vi "MEM Graph Holder.vi"(1 "Action(GET)":T5(ring), 7 "Mem Graph Ctl In":T1={"Chart Visible Time selector"=enum."1 minute", "Plot G1 L1"={"Var Tag"=0, "Color"=0, "Line Width"=0}, "Plot G1 L2"={"Var Tag"=0, "Color"=0, "Line Width"=0}, "Plot G1 R1"={"Var Tag"=0, "Color"=0, "Line Width"=0}, "Plot G1 R2"={"Var Tag"=0, "Color"=0, "Line Width"=0}, "Plot G2 L1"={"Var Tag"=0, "Color"=0, "Line Width"=0}, "Plot G2 L2"={"Var Tag"=0, "Color"=0, "Line Width"=0}, "Plot G2 R1"={"Var Tag"=0, "Color"=0, "Line Width"=0}, "Plot G2 R2"={"Var Tag"=0, "Color"=0, "Line Width"=0}, "G1 Y scale 0"={"Maximum"=0.0, "Minimum"=0.0, "Autoscaling"=0}, "G1 Y scale 1"={"Maximum"=0.0, "Minimum"=0.0, "Autoscaling"=0}, "G2 Y scale 0"={"Maximum"=0.0, "Minimum"=0.0, "Autoscaling"=0}, "G2 Y scale 1"={"Maximum"=0.0, "Minimum"=0.0, "Autoscaling"=0}} {"Plot G2 R2"."Line Width" items=["0", "1", "2", "3", "4", "5"]; "Plot G2 R2"."Var Tag" items=["", "Wire Length", "Wire Tension", "Wire Speed", "Topside Voltage", "Tool Head Voltage", "Current", "Resistance"]; "Plot G2 R1"."Line Width" items=["0", "1", "2", "3", "4", "5"]; "Plot G2 R1"."Var Tag" items=["", "Wire Length", "Wire Tension", "Wire Speed", "Topside Voltage", "Tool Head Voltage", "Current", "Resistance"]; "Plot G2 L2"."Line Width" items=["0", "1", "2", "3", "4", "5"]; "Plot G2 L2"."Var Tag" items=["", "Wire Length", "Wire Tension", "Wire Speed", "Topside Voltage", "Tool Head Voltage", "Current", "Resistance"]; "Plot G2 L1"."Line Width" items=["0", "1", "2", "3", "4", "5"]; "Plot G2 L1"."Var Tag" items=["", "Wire Length", "Wire Tension", "Wire Speed", "Topside Voltage", "Tool Head Voltage", "Current", "Resistance"]; "Plot G1 L1"."Line Width" items=["0", "1", "2", "3", "4", "5"]; "Plot G1 L1"."Var Tag" items=["", "Wire Length", "Wire Tension", "Wire Speed", "Topside Voltage", "Tool Head Voltage", "Current", "Resistance"]; "Plot G1 L2"."Line Width" items=["0", "1", "2", "3", "4", "5"]; "Plot G1 L2"."Var Tag" items=["", "Wire Length", "Wire Tension", "Wire Speed", "Topside Voltage", "Tool Head Voltage", "Current", "Resistance"]; "Plot G1 R2"."Line Width" items=["0", "1", "2", "3", "4", "5"]; "Plot G1 R2"."Var Tag" items=["", "Wire Length", "Wire Tension", "Wire Speed", "Topside Voltage", "Tool Head Voltage", "Current", "Resistance"]; "Plot G1 R1"."Line Width" items=["0", "1", "2", "3", "4", "5"]; "Plot G1 R1"."Var Tag" items=["", "Wire Length", "Wire Tension", "Wire Speed", "Topside Voltage", "Tool Head Voltage", "Current", "Resistance"]}, 11 "error in (no error)":errorcluster) -> (8 "Mem Graph Ctl Out":T1={"Chart Visible Time selector"=enum."1 minute", "Plot G1 L1"={"Var Tag"=0, "Color"=0, "Line Width"=0}, "Plot G1 L2"={"Var Tag"=0, "Color"=0, "Line Width"=0}, "Plot G1 R1"={"Var Tag"=0, "Color"=0, "Line Width"=0}, "Plot G1 R2"={"Var Tag"=0, "Color"=0, "Line Width"=0}, "Plot G2 L1"={"Var Tag"=0, "Color"=0, "Line Width"=0}, "Plot G2 L2"={"Var Tag"=0, "Color"=0, "Line Width"=0}, "Plot G2 R1"={"Var Tag"=0, "Color"=0, "Line Width"=0}, "Plot G2 R2"={"Var Tag"=0, "Color"=0, "Line Width"=0}, "G1 Y scale 0"={"Maximum"=0.0, "Minimum"=0.0, "Autoscaling"=0}, "G1 Y scale 1"={"Maximum"=0.0, "Minimum"=0.0, "Autoscaling"=0}, "G2 Y scale 0"={"Maximum"=0.0, "Minimum"=0.0, "Autoscaling"=0}, "G2 Y scale 1"={"Maximum"=0.0, "Minimum"=0.0, "Autoscaling"=0}} {"Plot G2 R2"."Line Width" items=["0", "1", "2", "3", "4", "5"]; "Plot G2 R2"."Var Tag" items=["", "Wire Length", "Wire Tension", "Wire Speed", "Topside Voltage", "Tool Head Voltage", "Current", "Resistance"]; "Plot G2 R1"."Line Width" items=["0", "1", "2", "3", "4", "5"]; "Plot G2 R1"."Var Tag" items=["", "Wire Length", "Wire Tension", "Wire Speed", "Topside Voltage", "Tool Head Voltage", "Current", "Resistance"]; "Plot G2 L2"."Line Width" items=["0", "1", "2", "3", "4", "5"]; "Plot G2 L2"."Var Tag" items=["", "Wire Length", "Wire Tension", "Wire Speed", "Topside Voltage", "Tool Head Voltage", "Current", "Resistance"]; "Plot G2 L1"."Line Width" items=["0", "1", "2", "3", "4", "5"]; "Plot G2 L1"."Var Tag" items=["", "Wire Length", "Wire Tension", "Wire Speed", "Topside Voltage", "Tool Head Voltage", "Current", "Resistance"]; "Plot G1 L1"."Line Width" items=["0", "1", "2", "3", "4", "5"]; "Plot G1 L1"."Var Tag" items=["", "Wire Length", "Wire Tension", "Wire Speed", "Topside Voltage", "Tool Head Voltage", "Current", "Resistance"]; "Plot G1 L2"."Line Width" items=["0", "1", "2", "3", "4", "5"]; "Plot G1 L2"."Var Tag" items=["", "Wire Length", "Wire Tension", "Wire Speed", "Topside Voltage", "Tool Head Voltage", "Current", "Resistance"]; "Plot G1 R2"."Line Width" items=["0", "1", "2", "3", "4", "5"]; "Plot G1 R2"."Var Tag" items=["", "Wire Length", "Wire Tension", "Wire Speed", "Topside Voltage", "Tool Head Voltage", "Current", "Resistance"]; "Plot G1 R1"."Line Width" items=["0", "1", "2", "3", "4", "5"]; "Plot G1 R1"."Var Tag" items=["", "Wire Length", "Wire Tension", "Wire Speed", "Topside Voltage", "Tool Head Voltage", "Current", "Resistance"]}, 15 "error out":errorcluster)   [LabVIEW 2011]
uses:
  Mem Graph Ctl Custer.ctl
  GUI/Shart Time Selector.ctl
  GUI/Graph/Plot selector.ctl
  GUI/Graph/Y scale cluster.ctl
  <vilib>/Utility/VariantDataType/VariantType.lvlib
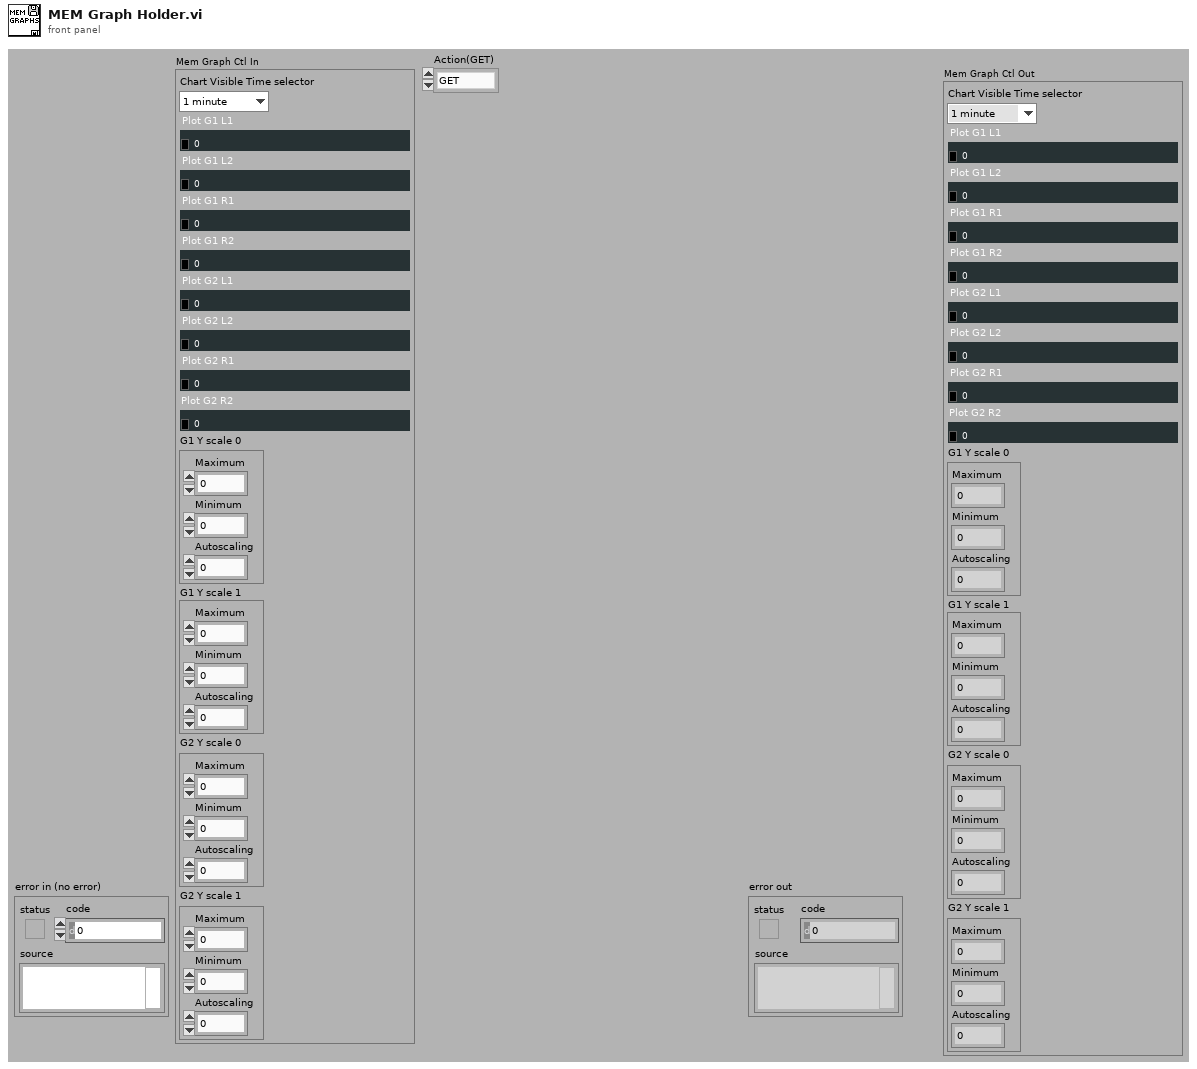
[diagram p1: front panel]
types:
  T1 = typedef "Mem Graph Ctl Custer.ctl" = cluster{"Chart Visible Time selector":T2, "Plot G1 L1":T3, "Plot G1 L2":T3, "Plot G1 R1":T3, "Plot G1 R2":T3, "Plot G2 L1":T3, "Plot G2 L2":T3, "Plot G2 R1":T3, "Plot G2 R2":T3, "G1 Y scale 0":T4, "G1 Y scale 1":T4, "G2 Y scale 0":T4, "G2 Y scale 1":T4}
  T2 = typedef "Shart Time Selector.ctl" = enum16{"10 Seconds", "1 minute", "5 minutes", "10 minutes", "30 minutes", "1 Hour"}
  T3 = typedef "Plot selector.ctl" = cluster{"Var Tag":u16, "Color":u32, "Line Width":u16}
  T4 = typedef "Y scale cluster.ctl" = cluster{"Maximum":dbl, "Minimum":dbl, "Autoscaling":i32}
  T5 = enum16{"GET", "SET", "Get from Ini", "Put in Ini"}
  T6 = typedef "List of tools.ctl" = enum16{"Stroker", "Driller", "Tractor"}
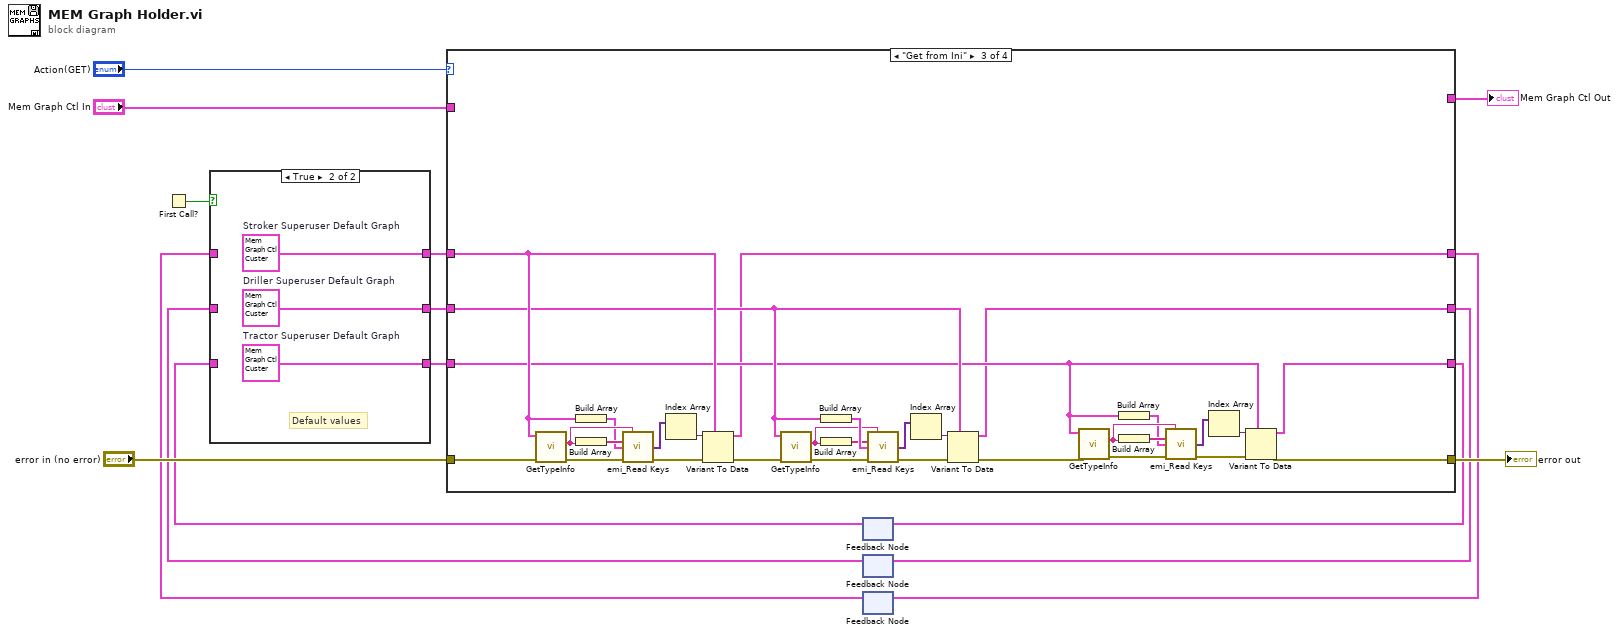
[diagram p0: block diagram]
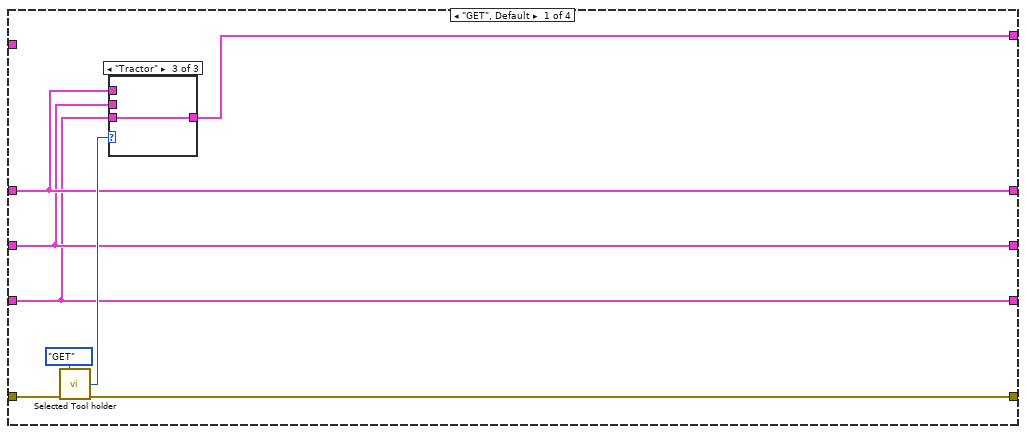
[diagram p3: hidden frame]
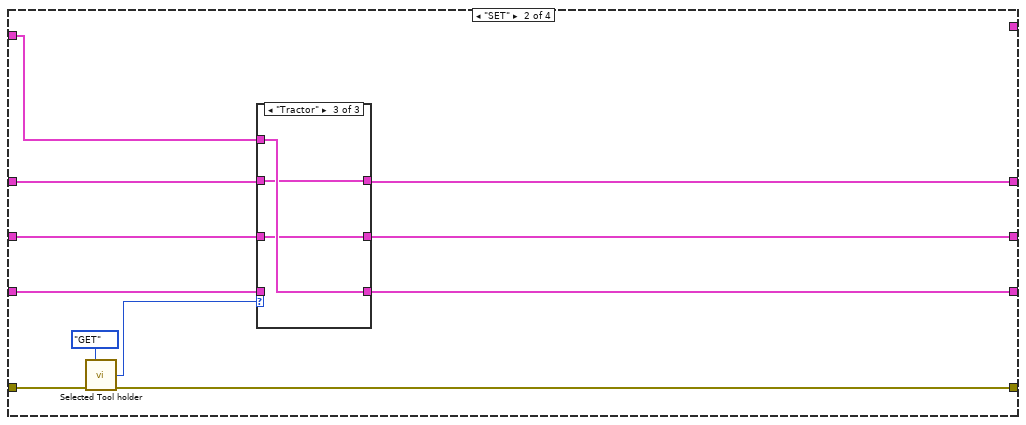
[diagram p6: hidden frame]
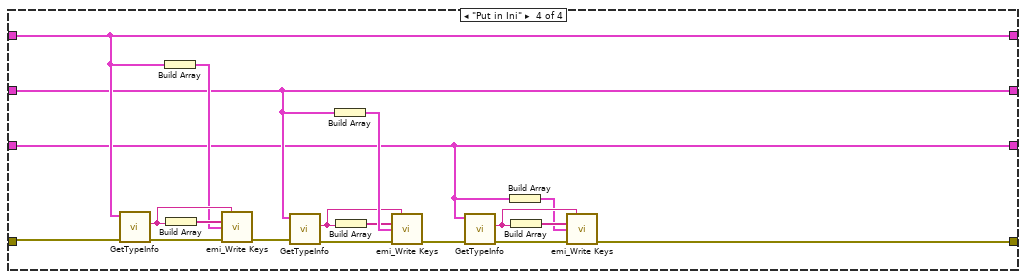
[diagram p9: hidden frame]
diagram:
  n1 = First Call?() -> (First Call?: T/F=w14:bool)
  n2 = feedback #1() -> (w1:T1)  [unwired: 1 in]
  n3 = feedback #2() -> (w2:T1)  [unwired: 1 in]
  n4 = feedback #3() -> (w3:T1)  [unwired: 1 in]
  n5 = case shown="True" w14 {
    tunnel: w3 -> [w18 _]
    tunnel: [w18 w21] -> w9
    tunnel: [w17 w20] -> w8
    tunnel: [w16 w19] -> w7
    tunnel: w2 -> [w17 _]
    tunnel: w1 -> [w16 _]
    frame False {
    }
    frame True {
      w19 = T1 {"Chart Visible Time selector"=enum."1 minute", "Plot G1 L1"={"Var Tag"=0, "Color"=16711680, "Line Width"=2}, "Plot G1 L2"={"Var Tag"=0, "Color"=16776960, "Line Width"=2}, "Plot G1 R1"={"Var Tag"=0, "Color"=16860, "Line Width"=2}, "Plot G1 R2"={"Var Tag"=0, "Color"=6618880, "Line Width"=2}, "Plot G2 L1"={"Var Tag"=0, "Color"=16711680, "Line Width"=2}, "Plot G2 L2"={"Var Tag"=0, "Color"=16776960, "Line Width"=2}, "Plot G2 R1"={"Var Tag"=0, "Color"=16860, "Line Width"=2}, "Plot G2 R2"={"Var Tag"=0, "Color"=6618880, "Line Width"=2}, "G1 Y scale 0"={"Maximum"=1.0, "Minimum"=-1.0, "Autoscaling"=0}, "G1 Y scale 1"={"Maximum"=1.0, "Minimum"=-1.0, "Autoscaling"=0}, "G2 Y scale 0"={"Maximum"=1.0, "Minimum"=-1.0, "Autoscaling"=0}, "G2 Y scale 1"={"Maximum"=1.0, "Minimum"=-1.0, "Autoscaling"=0}}  # Tractor Superuser Default Graph
      w20 = T1 {"Chart Visible Time selector"=enum."1 minute", "Plot G1 L1"={"Var Tag"=0, "Color"=16711680, "Line Width"=2}, "Plot G1 L2"={"Var Tag"=0, "Color"=16776960, "Line Width"=2}, "Plot G1 R1"={"Var Tag"=0, "Color"=16860, "Line Width"=2}, "Plot G1 R2"={"Var Tag"=0, "Color"=6618880, "Line Width"=2}, "Plot G2 L1"={"Var Tag"=0, "Color"=16711680, "Line Width"=2}, "Plot G2 L2"={"Var Tag"=0, "Color"=16776960, "Line Width"=2}, "Plot G2 R1"={"Var Tag"=0, "Color"=16860, "Line Width"=2}, "Plot G2 R2"={"Var Tag"=0, "Color"=6618880, "Line Width"=2}, "G1 Y scale 0"={"Maximum"=1.0, "Minimum"=-1.0, "Autoscaling"=0}, "G1 Y scale 1"={"Maximum"=1.0, "Minimum"=-1.0, "Autoscaling"=0}, "G2 Y scale 0"={"Maximum"=1.0, "Minimum"=-1.0, "Autoscaling"=0}, "G2 Y scale 1"={"Maximum"=1.0, "Minimum"=-1.0, "Autoscaling"=0}}  # Driller Superuser Default Graph
      w21 = T1 {"Chart Visible Time selector"=enum."1 minute", "Plot G1 L1"={"Var Tag"=0, "Color"=16711680, "Line Width"=2}, "Plot G1 L2"={"Var Tag"=0, "Color"=16776960, "Line Width"=2}, "Plot G1 R1"={"Var Tag"=0, "Color"=16860, "Line Width"=2}, "Plot G1 R2"={"Var Tag"=0, "Color"=6618880, "Line Width"=2}, "Plot G2 L1"={"Var Tag"=0, "Color"=16711680, "Line Width"=2}, "Plot G2 L2"={"Var Tag"=0, "Color"=16776960, "Line Width"=2}, "Plot G2 R1"={"Var Tag"=0, "Color"=16860, "Line Width"=2}, "Plot G2 R2"={"Var Tag"=0, "Color"=6618880, "Line Width"=2}, "G1 Y scale 0"={"Maximum"=1.0, "Minimum"=-1.0, "Autoscaling"=0}, "G1 Y scale 1"={"Maximum"=1.0, "Minimum"=-1.0, "Autoscaling"=0}, "G2 Y scale 0"={"Maximum"=1.0, "Minimum"=-1.0, "Autoscaling"=0}, "G2 Y scale 1"={"Maximum"=1.0, "Minimum"=-1.0, "Autoscaling"=0}}  # Stroker Superuser Default Graph
      # "Default values"
    }
  }
  n6 = case shown="\"Get from Ini\"" "Action(GET)" {
    tunnel: "error in (no error)" -> [w28 w35 w60 w88]
    tunnel: [w26 w34 w59 w87] -> w12
    tunnel: [w22 _ _ _] -> w10
    tunnel: "Mem Graph Ctl In" -> [_ w43 _ _]
    tunnel: w9 -> [w25 w42 w58 w86]
    tunnel: w8 -> [w24 w41 w57 w85]
    tunnel: w7 -> [w23 w40 w56 w84]
    tunnel: [w25 w37 w55 w86] -> w4
    tunnel: [w24 w38 w54 w85] -> w5
    tunnel: [w23 w39 w53 w84] -> w6
    frame "GET", Default {
      n7 = call "Selected Tool holder.vi"("Action(GET)"=enum16{"GET", "SET"}."GET", "error in (no error)"=w28) -> ("Tool out"=w27:T6, "error out"=w26:errorcluster)  [unwired: 12 in]
      n8 = case shown="\"Tractor\"" w27 {
        tunnel: w25 -> [w30 _ _]
        tunnel: w24 -> [_ w31 _]
        tunnel: w23 -> [_ _ w32]
        tunnel: [w30 w31 w32] -> w22
        frame "Stroker", Default {
        }
        frame "Driller" {
        }
        frame "Tractor" {
        }
      }
    }
    frame "SET" {
      n9 = call "Selected Tool holder.vi"("Action(GET)"=enum16{"GET", "SET"}."GET", "error in (no error)"=w35) -> ("Tool out"=w33:T6, "error out"=w34:errorcluster)  [unwired: 12 in]
      n10 = case shown="\"Tractor\"" w33 {
        tunnel: w43 -> [w46 w47 w52]
        tunnel: w40 -> [w44 w49 _]
        tunnel: w41 -> [w45 _ w51]
        tunnel: w42 -> [_ w48 w50]
        tunnel: [w45 w47 w51] -> w38
        tunnel: [w44 w49 w52] -> w39
        tunnel: [w46 w48 w50] -> w37
        frame "Stroker", Default {
        }
        frame "Driller" {
        }
        frame "Tractor" {
        }
      }
    }
    frame "Get from Ini" {
      n11 = call <vilib>:"GetTypeInfo.vi"("error in (no error)"=w60, "Variant"=w58) -> ("error out"=w64:errorcluster, "Name"=w65:string)  [unwired: 5 in, 3 out]
      n12 = Build Array(w58) -> (w61:T1[])
      n13 = Build Array(w65) -> (w62:string[])
      n14 = call "emi_Read Keys.vi"("Section"=w65, "Key Names"=w62, "Types/Defaults"=w61, "error in (no error)"=w64) -> ("Values"=w63:variant[], "error out"=w67:errorcluster)  [unwired: 9 in, 1 out]
      n15 = Index Array(array=w63) -> (element=w66:variant)  [unwired: 1 in]
      n16 = Variant To Data(error in=w67, type=w58, Variant=w66) -> (data=w55:T1, error out=w75:errorcluster)
      n17 = call <vilib>:"GetTypeInfo.vi"("error in (no error)"=w75, "Variant"=w57) -> ("error out"=w71:errorcluster, "Name"=w70:string)  [unwired: 5 in, 3 out]
      n18 = Build Array(w57) -> (w74:T1[])
      n19 = Build Array(w70) -> (w73:string[])
      n20 = call "emi_Read Keys.vi"("Section"=w70, "Key Names"=w73, "Types/Defaults"=w74, "error in (no error)"=w71) -> ("Values"=w72:variant[], "error out"=w68:errorcluster)  [unwired: 9 in, 1 out]
      n21 = Index Array(array=w72) -> (element=w69:variant)  [unwired: 1 in]
      n22 = Variant To Data(error in=w68, type=w57, Variant=w69) -> (data=w54:T1, error out=w83:errorcluster)
      n23 = call <vilib>:"GetTypeInfo.vi"("error in (no error)"=w83, "Variant"=w56) -> ("error out"=w79:errorcluster, "Name"=w80:string)  [unwired: 5 in, 3 out]
      n24 = Build Array(w56) -> (w76:T1[])
      n25 = Build Array(w80) -> (w77:string[])
      n26 = call "emi_Read Keys.vi"("Section"=w80, "Key Names"=w77, "Types/Defaults"=w76, "error in (no error)"=w79) -> ("Values"=w78:variant[], "error out"=w82:errorcluster)  [unwired: 9 in, 1 out]
      n27 = Index Array(array=w78) -> (element=w81:variant)  [unwired: 1 in]
      n28 = Variant To Data(error in=w82, type=w56, Variant=w81) -> (data=w53:T1, error out=w59:errorcluster)
    }
    frame "Put in Ini" {
      n29 = call <vilib>:"GetTypeInfo.vi"("error in (no error)"=w88, "Variant"=w86) -> ("error out"=w91:errorcluster, "Name"=w92:string)  [unwired: 5 in, 3 out]
      n30 = Build Array(w86) -> (w89:T1[])
      n31 = Build Array(w92) -> (w90:string[])
      n32 = call "emi_Write Keys.vi"("Section"=w92, "Key Names"=w90, "Values"=w89, "error in (no error)"=w91) -> ("error out"=w101:errorcluster)  [unwired: 10 in, 1 out]
      n33 = call <vilib>:"GetTypeInfo.vi"("error in (no error)"=w101, "Variant"=w85) -> ("error out"=w94:errorcluster, "Name"=w93:string)  [unwired: 5 in, 3 out]
      n34 = Build Array(w85) -> (w96:T1[])
      n35 = Build Array(w93) -> (w95:string[])
      n36 = call "emi_Write Keys.vi"("Section"=w93, "Key Names"=w95, "Values"=w96, "error in (no error)"=w94) -> ("error out"=w102:errorcluster)  [unwired: 10 in, 1 out]
      n37 = call <vilib>:"GetTypeInfo.vi"("error in (no error)"=w102, "Variant"=w84) -> ("error out"=w99:errorcluster, "Name"=w100:string)  [unwired: 5 in, 3 out]
      n38 = Build Array(w84) -> (w97:T1[])
      n39 = Build Array(w100) -> (w98:string[])
      n40 = call "emi_Write Keys.vi"("Section"=w100, "Key Names"=w98, "Values"=w97, "error in (no error)"=w99) -> ("error out"=w87:errorcluster)  [unwired: 10 in, 1 out]
    }
  }
  "error out" <- w12
  "Mem Graph Ctl Out" <- w10
  n41 = feedback-in #1(w6) -> ()
  n42 = feedback-in #2(w5) -> ()
  n43 = feedback-in #3(w4) -> ()
